vi "energyfeedback.vi"(7 "Magnet to Feedback":string="BTF/DHSTB002", 9 "X s [mm]":dbl=13.351557326910907 format="%.2f", 10 "X m [mm]":dbl format="%.2f", 11 "handleConnection":u32) -> (1 "lsee":bool, 2 "more":bool, 3 "feedback":bool, 4 "current set":dbl, 6 "current":dbl)   [LabVIEW 2014]
uses:
  common/crest/LabVIEW/LV14/libcommon-crest.lvlib
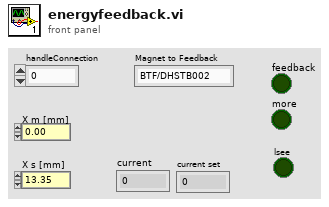
[diagram p1: front panel]
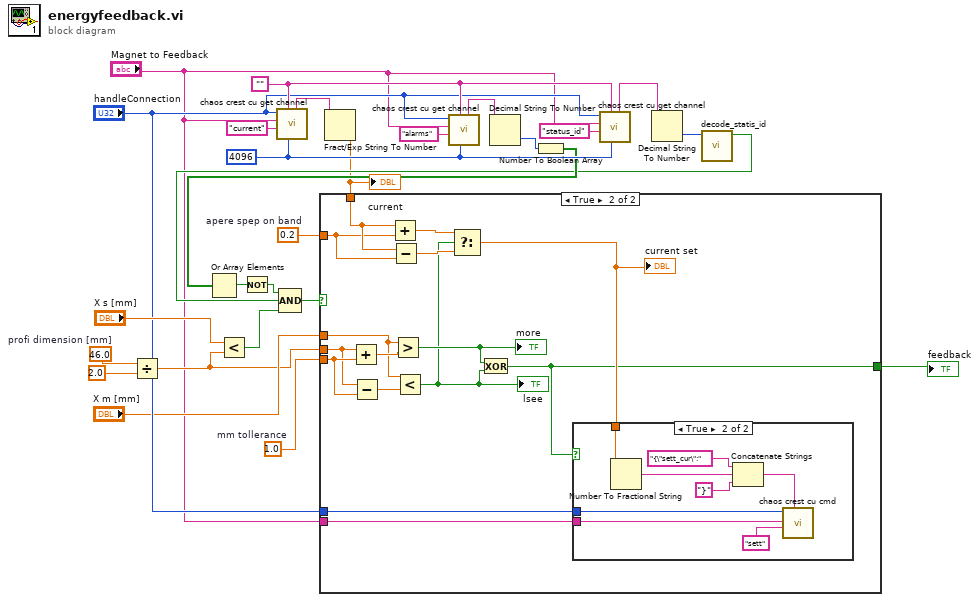
[diagram p0: block diagram]
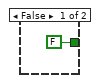
[diagram p2: hidden frame]
diagram:
  w4 = 1.0  # mm tollerance
  w6 = 0.2  # apere spep on band
  w12 = 46.0  # profi dimension [mm]
  w21 = "" ("value")
  w24 = 4096 ("maxsize")
  n1 = Divide(x=w12, y=2.0) -> (x/y=w2:dbl)
  n2 = Less?(x="X s [mm]", y=w2) -> (x < y?=w9:bool)
  n3 = call "chaos crest cu get channel.vi"("maxsize"=w24, "value"=w21, "channame"="current", "cuname"="Magnet to Feedback", "handleConnection"="handleConnection") -> ("value out"=w20:string)  [unwired: 5 in, 1 out]
  n4 = Fract/Exp String To Number(string=w20) -> (number=w7:dbl)  [unwired: 3 in, 1 out]
  "current" <- w7
  n5 = call "chaos crest cu get channel.vi"("maxsize"=w24, "value"=w21, "channame"="alarms", "cuname"="Magnet to Feedback", "handleConnection"="handleConnection") -> ("value out"=w19:string)  [unwired: 5 in, 1 out]
  n6 = Decimal String To Number(string=w19) -> (number=w18:i32)  [unwired: 2 in, 1 out]
  n7 = Number To Boolean Array(number=w18) -> (Boolean array=w16:bool[])
  n8 = Or Array Elements(Boolean array=w16) -> (logical OR=w17:bool)
  n9 = Not(x=w17) -> (.not. x?=w15:bool)
  n10 = call "chaos crest cu get channel.vi"("maxsize"=w24, "value"=w21, "channame"="status_id", "cuname"="Magnet to Feedback", "handleConnection"="handleConnection") -> ("value out"=w23:string)  [unwired: 5 in, 1 out]
  n11 = Decimal String To Number(string=w23) -> (number=w22:i32)  [unwired: 2 in, 1 out]
  n12 = call "decode_statis_id.vi"("satatus_id"=w22) -> ("Operational"=w14:bool)  [unwired: 7 in, 3 out]
  n13 = Compound Arithmetic op=AND(w15, w14, w9) -> (w13:bool)
  n14 = case shown="True" w13 {
    tunnel: "Magnet to Feedback" -> [_ w42]
    tunnel: "handleConnection" -> [_ w43]
    tunnel: w7 -> [_ w39]
    tunnel: w6 -> [_ w29]
    tunnel: "X m [mm]" -> [_ w32]
    tunnel: w4 -> [_ w36]
    tunnel: [FALSE w34] -> w3
    tunnel: w2 -> [_ w33]
    frame False {
    }
    frame True {
      n15 = Add(x=w33, y=w36) -> (x+y=w37:dbl)
      n16 = Subtract(x=w33, y=w36) -> (x-y=w35:dbl)
      n17 = Add(x=w39, y=w29) -> (x+y=w41:dbl)
      n18 = Subtract(x=w39, y=w29) -> (x-y=w38:dbl)
      n19 = Greater?(x=w32, y=w37) -> (0:w31:bool)
      "more" <- w31
      n20 = Less?(x=w32, y=w35) -> (x < y?=w30:bool)
      "lsee" <- w30
      n21 = Select(t=w41, s=w30, f=w38) -> (s? t:f=w40:dbl)
      "current set" <- w40
      n22 = Exclusive Or(1:w30, 2:w31) -> (0:w34:bool)
      n23 = case shown="True" w34 {
        tunnel: w43 -> [_ w46]
        tunnel: w42 -> [_ w45]
        tunnel: w40 -> [_ w44]
        frame False {
        }
        frame True {
          n24 = Number To Fractional String(number=w44) -> (F-format string=w49:string)  [unwired: 3 in]
          n25 = Concatenate Strings("{\"sett_cur\":", w49, "}" ("string")) -> (w48:string)
          n26 = call "chaos crest cu cmd.vi"("args"=w48, "cmd"="sett", "cuname"=w45, "handleConnection"=w46) -> ()  [unwired: 7 in, 1 out]
        }
      }
    }
  }
  "feedback" <- w3
